vi "command_builder.vi"(9 "Power Mode":T1(ring), 10 "Voltage/Current Mode":T2(ring), 11 "Variable":T3(ring)) -> (2 "Command out":string)   [LabVIEW 2015]
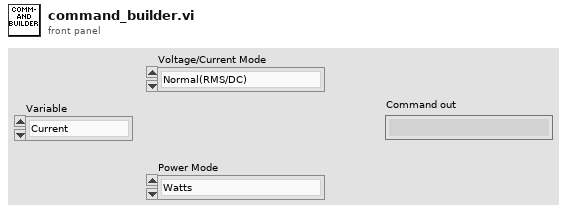
[diagram p1: front panel]
types:
  T1 = enum16{"Watts", "VA", "Power Factor", "Watts peak hold"}
  T2 = enum16{"Normal(RMS/DC)", "Peak", "Crest Factor", "Peak hold/Inrush (RMS/DC)"}
  T3 = enum16{"Current", "Voltage", "Power", "Frequency", "Curr,Volt, Power", "All"}
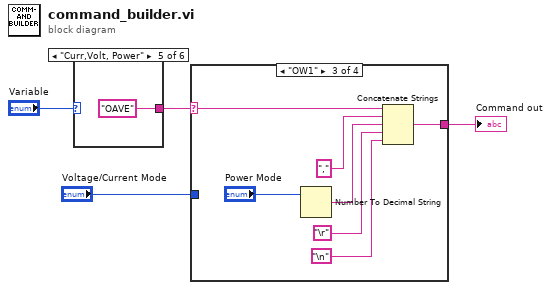
[diagram p0: block diagram]
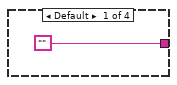
[diagram p2: hidden frame]
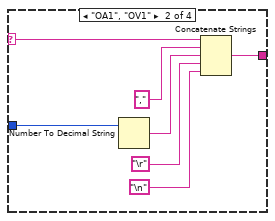
[diagram p3: hidden frame]
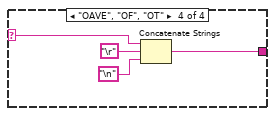
[diagram p4: hidden frame]
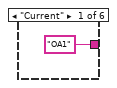
[diagram p5: hidden frame]
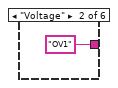
[diagram p6: hidden frame]
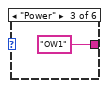
[diagram p7: hidden frame]
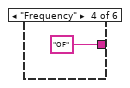
[diagram p8: hidden frame]
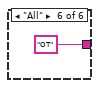
[diagram p9: hidden frame]
diagram:
  n1 = case shown="\"Curr,Volt, Power\"" "Variable" {
    tunnel: ["OA1" "OV1" "OW1" "OF" "OAVE" "OT"] -> w3
    frame "Current" {
    }
    frame "Voltage" {
    }
    frame "Power" {
    }
    frame "Frequency" {
    }
    frame "Curr,Volt, Power" {
    }
    frame "All" {
    }
  }
  n2 = case shown="\"OW1\"" w3 {
    selector: w3 -> [_ w13 w20 w29]
    tunnel: "Voltage/Current Mode" -> [_ w14 _ _]
    tunnel: ["" w12 w21 w28] -> w1
    frame Default {
    }
    frame "OA1", "OV1" {
      n3 = Number To Decimal String(number=w14) -> (decimal integer string=w15:string)  [unwired: 1 in]
      n4 = Concatenate Strings(w13, "," ("string"), w15, "\r", "\n") -> (w12:string)
    }
    frame "OW1" {
      n5 = Number To Decimal String(number="Power Mode") -> (decimal integer string=w22:string)  [unwired: 1 in]
      n6 = Concatenate Strings(w20, "," ("string"), w22, "\r", "\n") -> (w21:string)
    }
    frame "OAVE", "OF", "OT" {
      n7 = Concatenate Strings(w29, "\r", "\n") -> (w28:string)
    }
  }
  "Command out" <- w1
